vi "Teleop.vi"(10 "Match Info":T1={"Autonomous Elapsed Seconds"=0.0, "TeleOp Elapsed Seconds"=0.0, "Disabled Elapsed Seconds"=0.0, "Visited Autonomous"=FALSE, "Visited TeleOp"=FALSE, "Visited Disabled"=FALSE, "Autonomous Settings"={"Autonomous Style"=enum."Independent", "VI Refnum"=refnum}}, 11 "Call Context":T2) -> ()   [LabVIEW 2019]
doc: "This VI is called for each TeleOp packet received from the DS where the robot is not disabled. It is often used to read from the joysticks and update I/O or to update setpoints for timed control loops. It should complete and return within 20 milliseconds or it may miss DS packets."
uses:
  <vilib>/Rock Robotics/WPI/DriverStation/WPI_DriverStationDerivedRobotMode.ctl
  <vilib>/Rock Robotics/WPI/DriverStation/WPI_DriverStationMatch Info.ctl
  <vilib>/Rock Robotics/WPI/DriverStation/WPI_DriverStationRobotMode2.ctl
  <vilib>/Rock Robotics/WPI/ThirdParty/REV Robotics/SPARK MAX/Typedef/Spark MAX Control Type.ctl
  <vilib>/Rock Robotics/WPI/Utilities/WPI_GetSetVariantRefNum.vi
  Robot Global Data.vi
  <vilib>/Rock Robotics/Network Tables/NT Write Number.vi
  <vilib>/Rock Robotics/Network Tables/NT Write Boolean.vi
  <vilib>/Rock Robotics/WPI/RobotDrive/WPI_RobotDriveArcadeDrive_Standard(NoSaturation).vi
  <vilib>/Rock Robotics/Network Tables/NT Write Numeric Array.vi
panel:
  in  "error in":errorcluster
  # "Click here to set min"
  # "Click here to set max"
  # "Click here to set min"
  # "Click here to set max"
  # "Click here to set min"
  # "Click here to set max"
  # "Click here to set min"
  # "Click here to set max"
  # "Click here to set min"
  # "Click here to set max"
  # "Click here to set min"
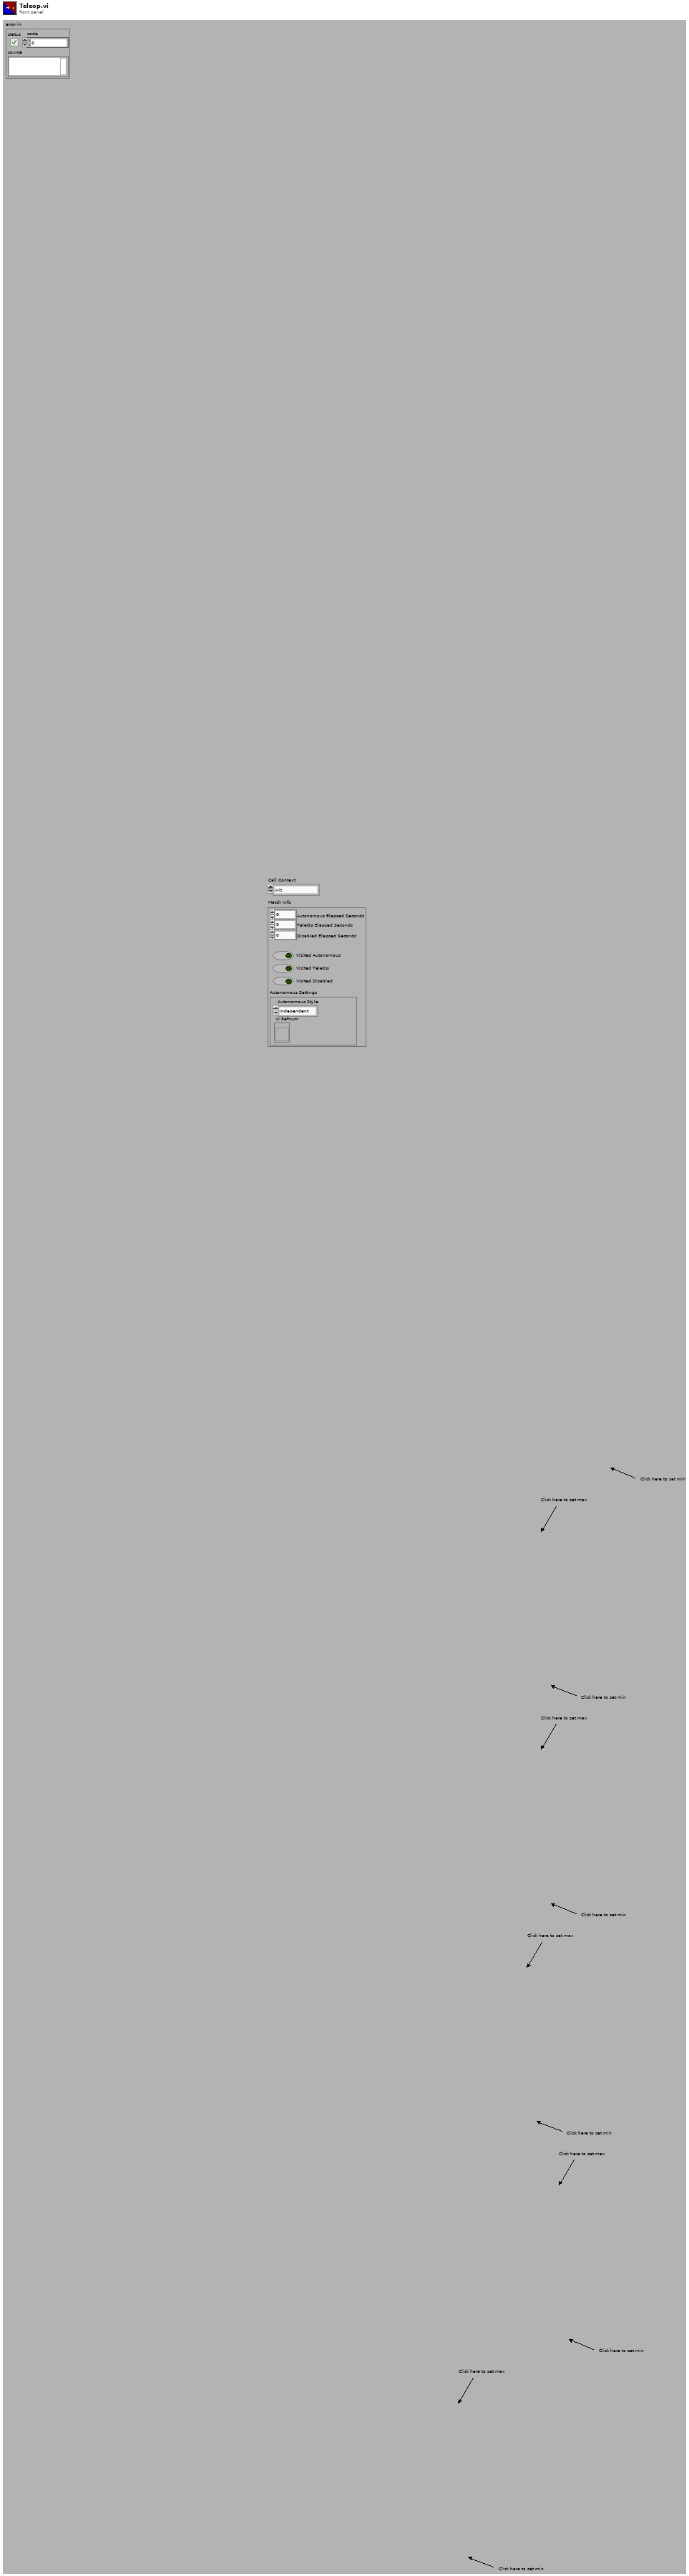
[diagram p1: front panel]
types:
  T1 = typedef "WPI_DriverStationMatch Info.ctl" = cluster{"Autonomous Elapsed Seconds":dbl, "TeleOp Elapsed Seconds":dbl, "Disabled Elapsed Seconds":dbl, "Visited Autonomous":bool, "Visited TeleOp":bool, "Visited Disabled":bool, "Autonomous Settings":cluster{"Autonomous Style":enum16{"Iterative", "Independent"}, "VI Refnum":refnum<vi>}}
  T2 = typedef "WPI_DriverStationDerivedRobotMode.ctl" = enum16{"Init", "Execute", "Stop"}
  T3 = typedef "WPI_JoystickDevRef.ctl" = cluster{"Device":T4}
  T4 = typedef "WPI_JoystickDeviceEnum.ctl" = enum16{"USB 0", "USB 1", "USB 2", "USB 3", "USB 4", "USB 5"}
  T5 = typedef "WPI_MotorControlDeviceRef.ctl" = cluster{"DeviceStatus":errorcluster, "Type":T6, "PWM":cluster{"PWM Channel":T7, "DeadBand":T8}, "CAN":cluster{"Device Number":u8, "SetOutput VI Ref":variant, "GetOutput VI Ref":variant, "Enable VI Ref":variant, "Disable VI Ref":variant, "Data":variant}, "Invert":bool, "DIO PWM":cluster{"PWM \"Enable\" Channel":T7, "DIOChannel":T9, "PWM Rate":dbl}}
  T6 = typedef "WPI_MotorControlType.ctl" = enum16{"PWM", "CAN", "DIO PWM"}
  T7 = typedef "FPGA_DIOPWMChannel.ctl" = enum8{"PWM 0", "PWM 1", "PWM 2", "PWM 3", "PWM 4", "PWM 5", "PWM 6", "PWM 7", "PWM 8", "PWM 9", "PWM MXP 0", "PWM MXP 1", "PWM MXP 2", "PWM MXP 3", "PWM MXP 4", "PWM MXP 5", "PWM MXP 6", "PWM MXP 7", "PWM MXP 8", "PWM MXP 9", "Invalid"}
  T8 = typedef "WPI_PWMDeadband.ctl" = cluster{"Name":string, "maxPositivePwm":i32, "minPositivePwm":i32, "centerPwm":i32, "maxNegativePwm":i32, "minNegativePwm":i32, "angularRange":u16}
  T9 = typedef "FPGA_DIOChannel.ctl" = enum8{"DIO 0", "DIO 1", "DIO 2", "DIO 3", "DIO 4", "DIO 5", "DIO 6", "DIO 7", "DIO 8", "DIO 9", "DIO MXP 0", "DIO MXP 1", "DIO MXP 2", "DIO MXP 3", "DIO MXP 4", "DIO MXP 5", "DIO MXP 6", "DIO MXP 7", "DIO MXP 8", "DIO MXP 9", "DIO MXP 10", "DIO MXP 11", "DIO MXP 12", "DIO MXP 13", "DIO MXP 14", "DIO MXP 15", "SPI Port CS1", "SPI Port CS2", "SPI Port CS3", "SPI Port MISO", "SPI Port MOSI", "Invalid"}
  T10 = typedef "WPI_RobotDriveDevRef.ctl" = cluster{"DevStatus":errorcluster, "Motors[]":T5[], "Square Inputs":bool, "Max Output":dbl}
  T11 = typedef "WPI_ServoDeviceRef.ctl" = cluster{"DeviceStatus":errorcluster, "PWM Channel":T7, "DeadBand":T8}
  T12 = typedef "Spark MAX Control Type.ctl" = enum16{"Percent VBus", "Voltage", "Velocity", "Position", "Smart Motion", "Current", "Smart Velocity"}
  T13 = typedef "WPI_DriverStationRobotMode2.ctl" = enum16{"Autonomous Disabled", "Autonomous Enabled", "Teleop Disabled", "Teleop Enabled", "Disconnected", "Finish", "Test Disabled", "Test Enabled", "Emergency Stopped"}
  T14 = cluster{"P Gain":dbl, "I Gain":dbl, "D Gain":dbl, "F Gain":dbl, "I Zone":dbl, "Min Output":dbl, "Max Output":dbl}
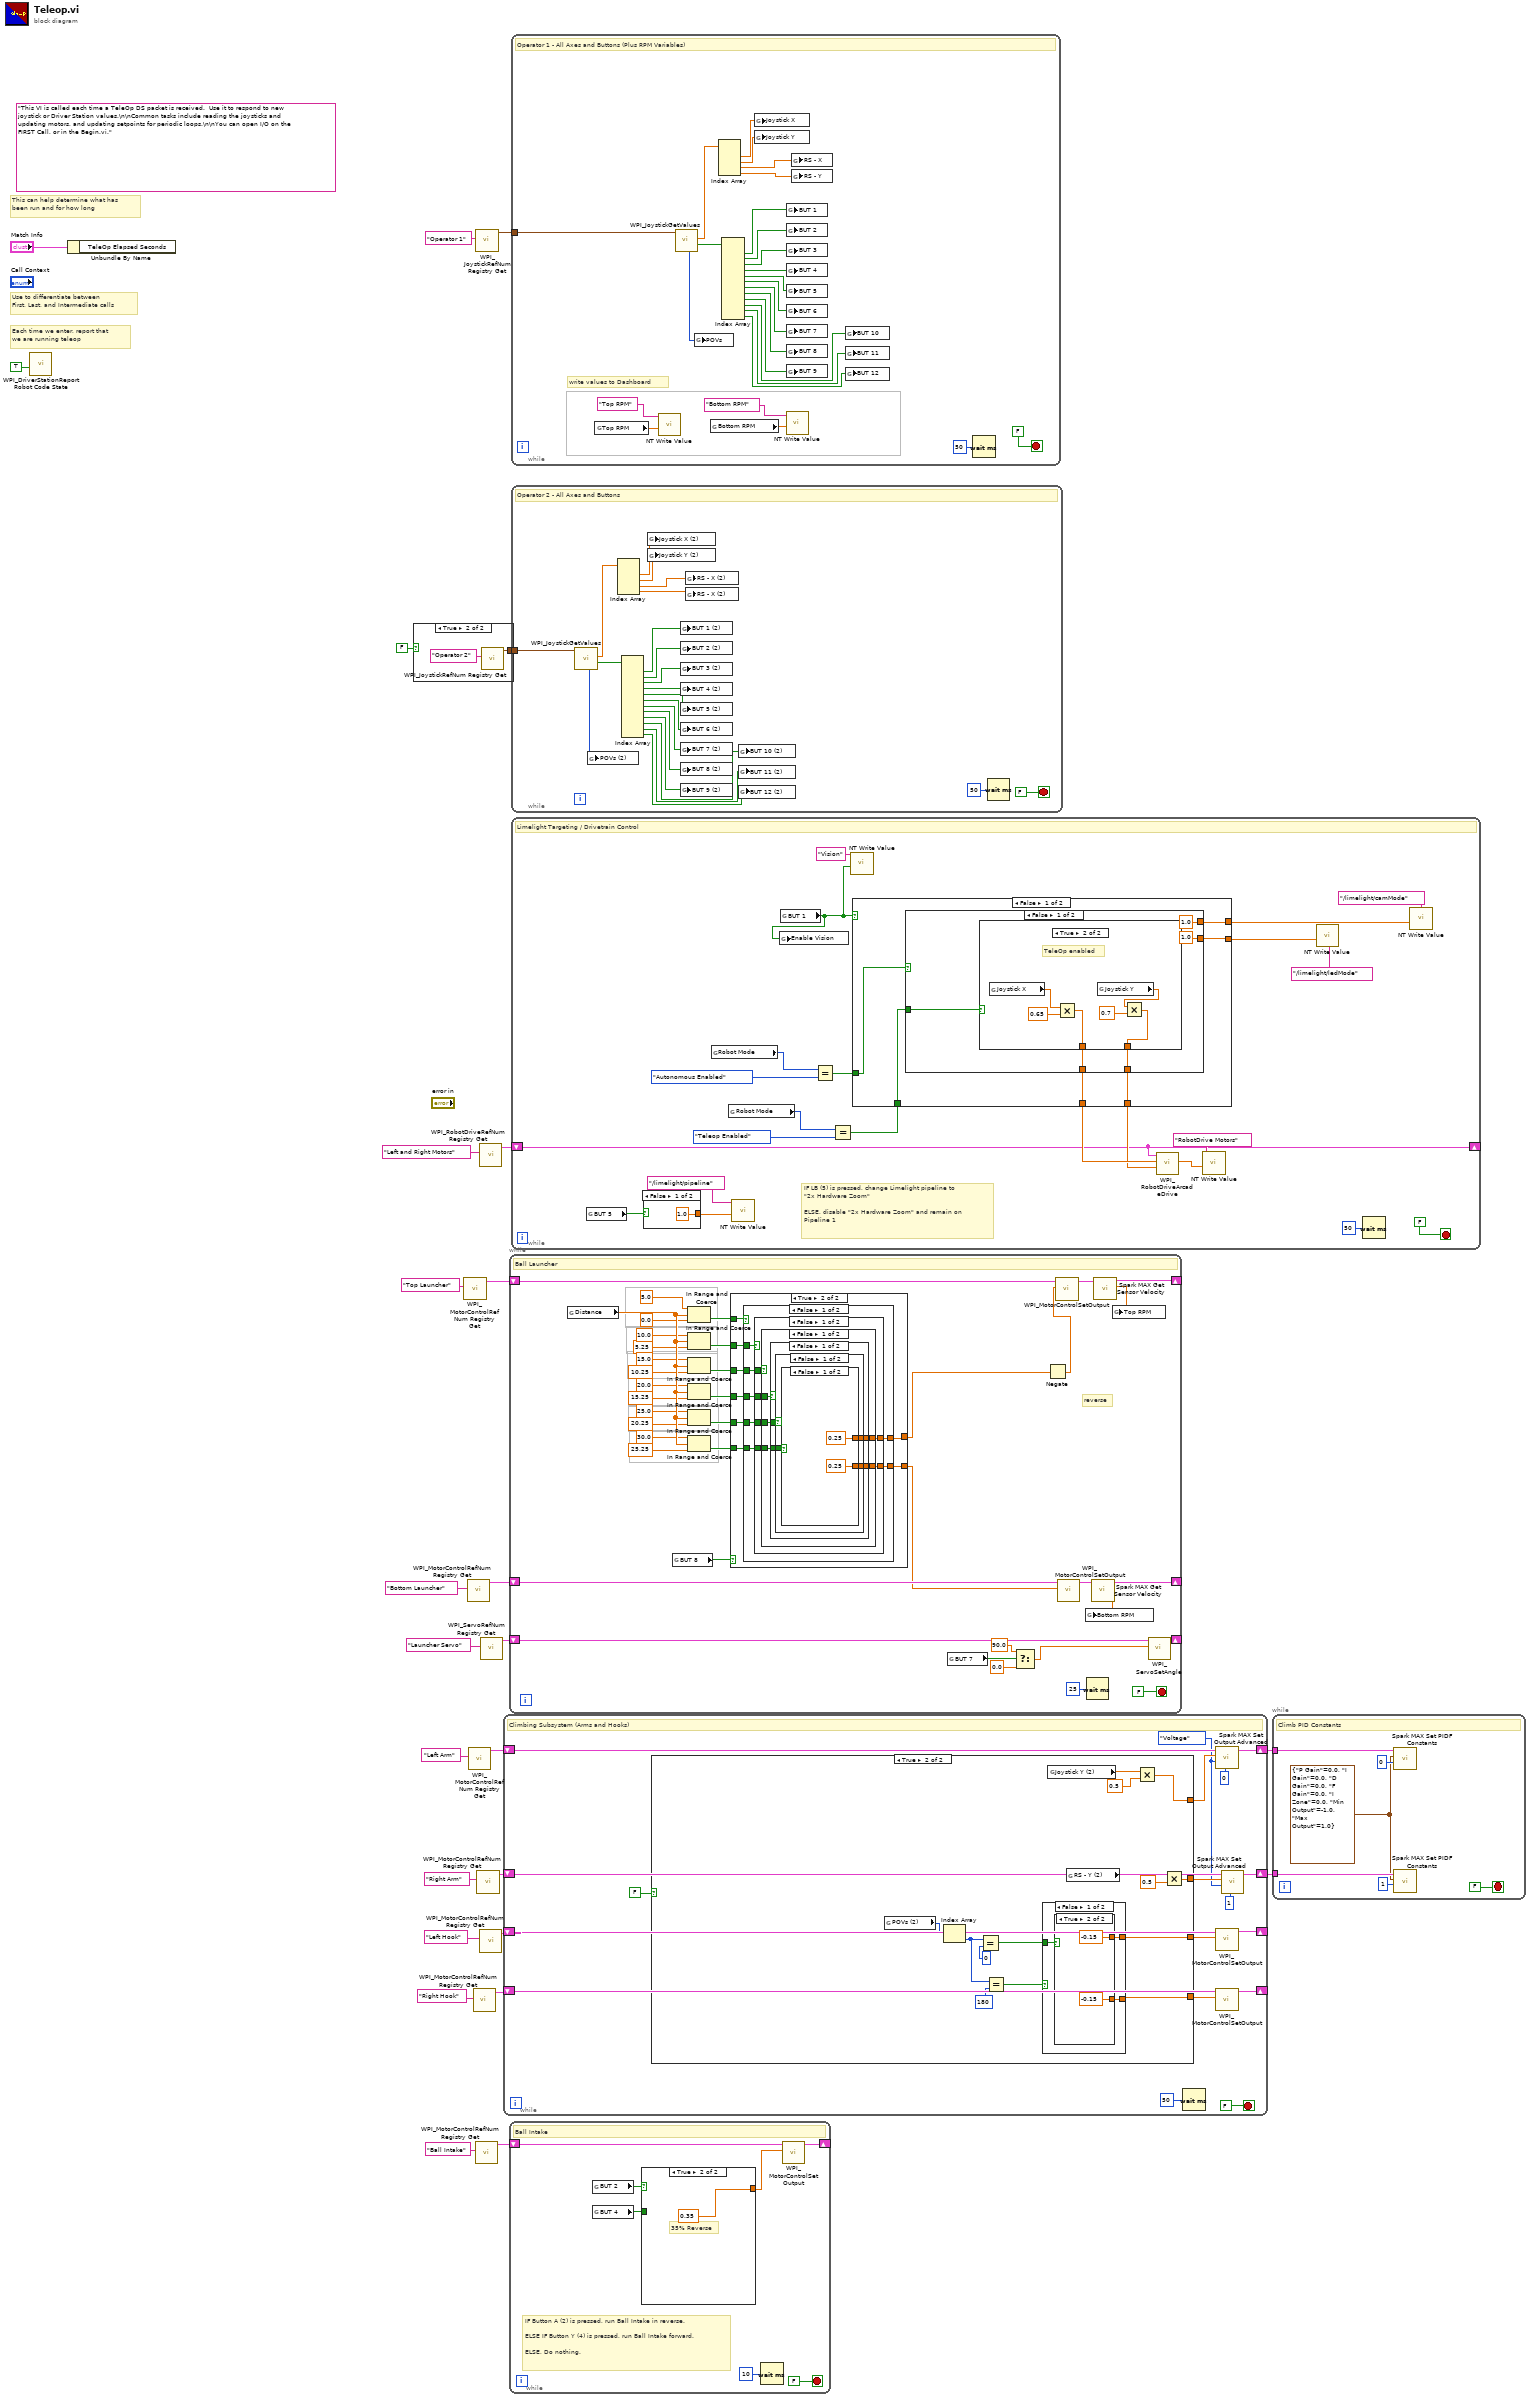
[diagram p0: block diagram]
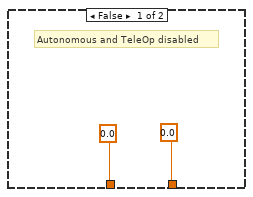
[diagram p3: hidden frame]
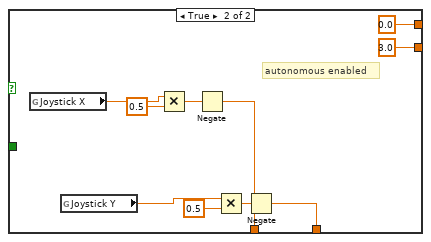
[diagram p4: hidden frame]
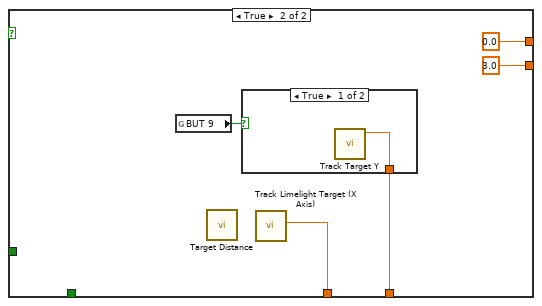
[diagram p5: hidden frame]
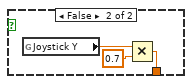
[diagram p6: hidden frame]
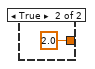
[diagram p7: hidden frame]
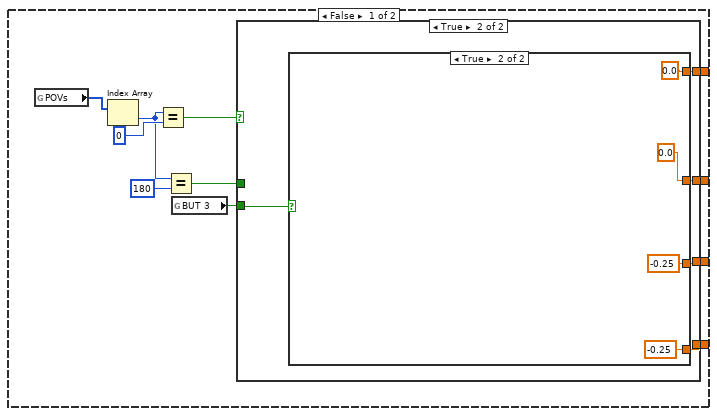
[diagram p8: hidden frame]
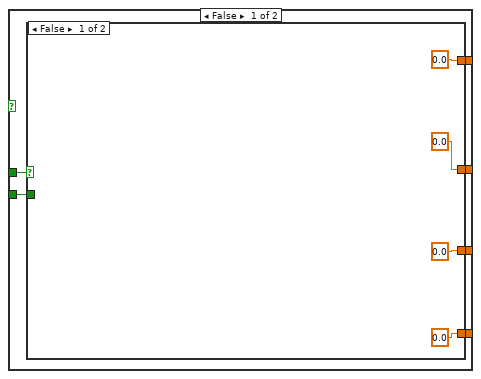
[diagram p9: hidden frame]
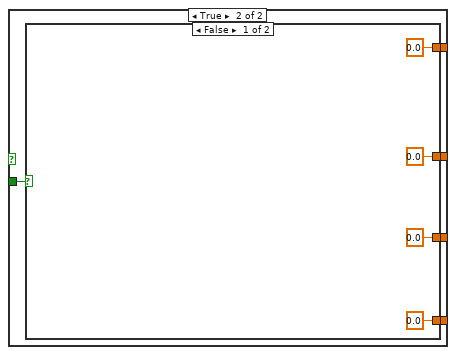
[diagram p10: hidden frame]
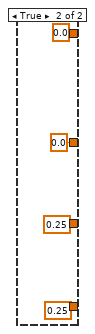
[diagram p11: hidden frame]
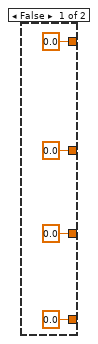
[diagram p12: hidden frame]
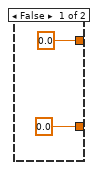
[diagram p13: hidden frame]
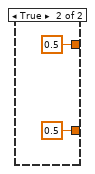
[diagram p14: hidden frame]
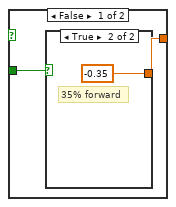
[diagram p15: hidden frame]
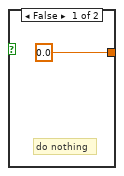
[diagram p16: hidden frame]
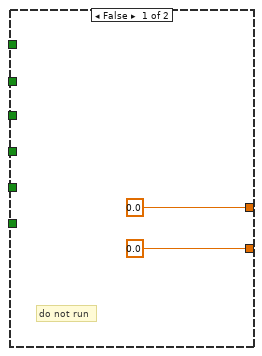
[diagram p17: hidden frame]
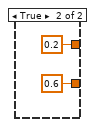
[diagram p18: hidden frame]
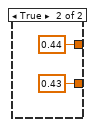
[diagram p19: hidden frame]
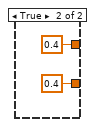
[diagram p20: hidden frame]
diagram:
  (unwired) "This VI is called each time a TeleOp DS packet is received.  Use it to respond to new joystick or Driver Station values.\n\nCommon tasks include reading the joysticks and updating motors, and updating setpoints for periodic loops.\n\nYou can open I/O on the FIRST Call, or in the Begin.vi."
  # "Each time we enter, report that\nwe are running teleop"
  # "Use to differentiate between\nFirst, Last, and Intermediate calls"
  # "This can help determine what has\nbeen run and for how long"
  n1 = call <vilib>:"WPI_DriverStationReport Robot Code State.vi"("TeleOp"=TRUE ("Autonomous")) -> ()  [unwired: 10 in, 1 out]
  n2 = Unbundle By Name("Match Info") -> ()  [unwired: 1 out]
  n3 = case shown="True" FALSE {
    tunnel: [_ w27] -> w8
    frame False {
    }
    frame True {
      n4 = call <vilib>:"WPI_JoystickRefNum Registry Get.vi"("refnum name"="Operator 2") -> ("JoystickDevRef"=w27:T3)  [unwired: 1 in, 9 out]
    }
  }
  n5 = call <vilib>:"WPI_MotorControlRefNum Registry Get.vi"("refnum name"="Top Launcher") -> ("MotorControlDevRef"=w20:T5)  [unwired: 9 in, 1 out]
  n6 = call <vilib>:"WPI_MotorControlRefNum Registry Get.vi"("refnum name"="Bottom Launcher") -> ("MotorControlDevRef"=w22:T5)  [unwired: 9 in, 1 out]
  n7 = call <vilib>:"WPI_MotorControlRefNum Registry Get.vi"("refnum name"="Left Arm") -> ("MotorControlDevRef"=w14:T5)  [unwired: 9 in, 1 out]
  n8 = call <vilib>:"WPI_MotorControlRefNum Registry Get.vi"("refnum name"="Right Hook") -> ("MotorControlDevRef"=w11:T5)  [unwired: 9 in, 1 out]
  n9 = call <vilib>:"WPI_MotorControlRefNum Registry Get.vi"("refnum name"="Ball Intake") -> ("MotorControlDevRef"=w16:T5)  [unwired: 9 in, 1 out]
  n10 = call <vilib>:"WPI_JoystickRefNum Registry Get.vi"("refnum name"="Operator 1") -> ("JoystickDevRef"=w7:T3)  [unwired: 1 in, 9 out]
  n11 = call <vilib>:"WPI_MotorControlRefNum Registry Get.vi"("refnum name"="Right Arm") -> ("MotorControlDevRef"=w13:T5)  [unwired: 9 in, 1 out]
  n12 = call <vilib>:"WPI_RobotDriveRefNum Registry Get.vi"("refnum name"="Left and Right Motors") -> ("RobotDriveDevRef"=w1:T10)  [unwired: 1 in, 9 out]
  n13 = call <vilib>:"WPI_MotorControlRefNum Registry Get.vi"("refnum name"="Left Hook") -> ("MotorControlDevRef"=w12:T5)  [unwired: 9 in, 1 out]
  n14 = call <vilib>:"WPI_ServoRefNum Registry Get.vi"("refnum name"="Launcher Servo") -> ("ServoDeviceRef"=w18:T11)  [unwired: 9 in, 1 out]
  n15 = while {
    shift-right: [w45] -> w3
    shift-left: w14 -> [w44]
    shift-right: [w33] -> w2
    shift-left: w13 -> [w32]
    shift-right: [w41] -> _
    shift-left: w11 -> [w40]
    shift-right: [w42] -> _
    shift-left: w12 -> [w39]
    stop <- FALSE stop-if-true
    w29 = Spark_MAX_Control_Type."Voltage" ("Control Mode")
    # "Climbing Subsystem (Arms and Hooks)"
    n16 = case shown="True" FALSE {
      tunnel: [w56 w107] -> w38
      tunnel: [w57 w106] -> w37
      tunnel: [w54 w100] -> w36
      tunnel: [w55 w99] -> w31
      frame False {
        n17 = global read "Robot Global Data.vi" "POVs"() -> (w53:i16[])
        n18 = Index Array(array=w53) -> (element=w51:i16)  [unwired: 1 in]
        n19 = Equal?(x=w51, y=i16 0) -> (x = y?=w49:bool)
        n20 = Equal?(x=w51, y=i16 180) -> (x = y?=w48:bool)
        n21 = global read "Robot Global Data.vi" "BUT 3"() -> (w47:bool)
        n22 = case shown="True" w49 {
          tunnel: [w63 w82] -> w57
          tunnel: [w62 w81] -> w56
          tunnel: [w61 w83] -> w55
          tunnel: [w60 w84] -> w54
          tunnel: w48 -> [w59 _]
          tunnel: w47 -> [w58 w85]
          frame False {
            n23 = case shown="False" w59 {
              tunnel: [0.0 ("Output") w72] -> w63
              tunnel: [0.0 ("Output") w71] -> w62
              tunnel: [0.0 w70] -> w61
              tunnel: [0.0 w69] -> w60
              tunnel: w58 -> [_ w68]
              frame False {
              }
              frame True {
                n24 = case shown="False" w68 {
                  tunnel: [0.0 ("Output") 0.25 ("Output")] -> w72
                  tunnel: [0.0 ("Output") 0.25 ("Output")] -> w71
                  tunnel: [0.0 0.0] -> w70
                  tunnel: [0.0 0.0] -> w69
                  frame False {
                  }
                  frame True {
                  }
                }
              }
            }
          }
          frame True {
            n25 = case shown="True" w85 {
              tunnel: [0.0 0.0] -> w84
              tunnel: [0.0 0.0] -> w83
              tunnel: [0.0 ("Output") -0.25 ("Output")] -> w82
              tunnel: [0.0 ("Output") -0.25 ("Output")] -> w81
              frame False {
              }
              frame True {
              }
            }
          }
        }
      }
      frame True {
        n26 = global read "Robot Global Data.vi" "POVs (2)"() -> (w105:i16[])
        n27 = Index Array(array=w105) -> (element=w104:i16)  [unwired: 1 in]
        n28 = Equal?(x=w104, y=i16 0) -> (x = y?=w101:bool)
        n29 = Equal?(x=w104, y=i16 180) -> (x = y?=w102:bool)
        n30 = case shown="False" w102 {
          tunnel: [w110 0.5 ("Output")] -> w107
          tunnel: [w109 0.5 ("Output")] -> w106
          tunnel: w101 -> [w108 _]
          frame False {
            n31 = case shown="True" w108 {
              tunnel: [0.0 ("Output") -0.15 ("Output")] -> w110
              tunnel: [0.0 ("Output") -0.15 ("Output")] -> w109
              frame False {
              }
              frame True {
              }
            }
          }
          frame True {
          }
        }
        n32 = global read "Robot Global Data.vi" "Joystick Y (2)"() -> (w98:dbl)
        n33 = global read "Robot Global Data.vi" "RS - Y (2)"() -> (w97:dbl)
        n34 = Multiply(x=w98, y=0.5) -> (x*y=w100:dbl)
        n35 = Multiply(x=w97, y=0.5) -> (x*y=w99:dbl)
      }
    }
    n36 = Wait (ms)(milliseconds to wait=u32 50) -> ()  [unwired: 1 out]
    n37 = call <vilib>:"Spark MAX Set Output Advanced.vi"("PIDF Slot (0)"=0, "Control Mode"=w29, "Setpoint"=w36, "MotorControlDevRef"=w44) -> ("MotorControlDevRef"=w45:T5)  [unwired: 6 in, 1 out]
    n38 = call <vilib>:"WPI_MotorControlSetOutput.vi"("Output"=w37, "MotorControlDevRef"=w39) -> ("MotorControlDevRef"=w42:T5)  [unwired: 7 in, 2 out]
    n39 = call <vilib>:"WPI_MotorControlSetOutput.vi"("Output"=w38, "MotorControlDevRef"=w40) -> ("MotorControlDevRef"=w41:T5)  [unwired: 7 in, 2 out]
    n40 = call <vilib>:"Spark MAX Set Output Advanced.vi"("PIDF Slot (0)"=1, "Control Mode"=w29, "Setpoint"=w31, "MotorControlDevRef"=w32) -> ("MotorControlDevRef"=w33:T5)  [unwired: 6 in, 1 out]
  }
  n41 = while {
    shift-right: [w147] -> _
    shift-left: w22 -> [w148]
    shift-right: [w145] -> _
    shift-left: w20 -> [w146]
    shift-right: [w144] -> _
    shift-left: w18 -> [w139]
    stop <- FALSE stop-if-true
    # "reverse"
    # "Ball Launcher"
    n42 = global read "Robot Global Data.vi" "Distance"() -> (w138:dbl)
    n43 = global read "Robot Global Data.vi" "BUT 8"() -> (w119:bool)
    n44 = In Range and Coerce(upper limit=5.0, x=w138, lower limit=0.0) -> (In Range?=w137:bool)  [unwired: 1 out]
    n45 = In Range and Coerce(upper limit=10.0, x=w138, lower limit=5.25) -> (In Range?=w136:bool)  [unwired: 1 out]
    n46 = In Range and Coerce(upper limit=15.0, x=w138, lower limit=10.25) -> (In Range?=w120:bool)  [unwired: 1 out]
    n47 = In Range and Coerce(upper limit=20.0, x=w138, lower limit=15.25) -> (In Range?=w121:bool)  [unwired: 1 out]
    n48 = In Range and Coerce(upper limit=25.0, x=w138, lower limit=20.25) -> (In Range?=w122:bool)  [unwired: 1 out]
    n49 = In Range and Coerce(upper limit=30.0, x=w138, lower limit=25.25) -> (In Range?=w123:bool)  [unwired: 1 out]
    n50 = case shown="True" w119 {
      tunnel: [0.0 ("Output") w159] -> w118
      tunnel: [0.0 ("Output") w158] -> w117
      tunnel: w137 -> [_ w165]
      tunnel: w120 -> [_ w163]
      tunnel: w121 -> [_ w162]
      tunnel: w122 -> [_ w161]
      tunnel: w123 -> [_ w160]
      tunnel: w136 -> [_ w164]
      frame False {
        # "do not run"
      }
      frame True {
        n51 = case shown="False" w165 {
          tunnel: w164 -> [w172 _]
          tunnel: w163 -> [w171 _]
          tunnel: w162 -> [w170 _]
          tunnel: w161 -> [w169 _]
          tunnel: w160 -> [w168 _]
          tunnel: [w167 0.0 ("Output")] -> w159
          tunnel: [w166 0.0 ("Output")] -> w158
          frame False {
            n52 = case shown="False" w172 {
              tunnel: w171 -> [w178 _]
              tunnel: w170 -> [w177 _]
              tunnel: w169 -> [w176 _]
              tunnel: w168 -> [w175 _]
              tunnel: [w174 0.4 ("Output")] -> w167
              tunnel: [w173 0.65 ("Output")] -> w166
              frame False {
                n53 = case shown="False" w178 {
                  tunnel: w177 -> [w183 _]
                  tunnel: w176 -> [w182 _]
                  tunnel: w175 -> [w181 _]
                  tunnel: [w180 0.3 ("Output")] -> w174
                  tunnel: [w179 0.55 ("Output")] -> w173
                  frame False {
                    n54 = case shown="False" w183 {
                      tunnel: w182 -> [w187 _]
                      tunnel: w181 -> [w186 _]
                      tunnel: [w185 0.4 ("Output")] -> w180
                      tunnel: [w184 0.4 ("Output")] -> w179
                      frame False {
                        n55 = case shown="False" w187 {
                          tunnel: w186 -> [w190 _]
                          tunnel: [w189 0.44 ("Output")] -> w185
                          tunnel: [w188 0.43 ("Output")] -> w184
                          frame False {
                            n56 = case shown="False" w190 {
                              tunnel: [0.25 ("Output") 0.2 ("Output")] -> w189
                              tunnel: [0.25 ("Output") 0.6 ("Output")] -> w188
                              frame False {
                              }
                              frame True {
                              }
                            }
                          }
                          frame True {
                          }
                        }
                      }
                      frame True {
                      }
                    }
                  }
                  frame True {
                  }
                }
              }
              frame True {
              }
            }
          }
          frame True {
            # "do not run"
          }
        }
      }
    }
    n57 = global read "Robot Global Data.vi" "BUT 7"() -> (w143:bool)
    n58 = Select(t=90.0, s=w143, f=0.0) -> (s? t:f=w140:dbl)
    n59 = Negate(x=w118) -> (-x=w155:dbl)
    n60 = call <vilib>:"WPI_MotorControlSetOutput.vi"("Output"=w155, "MotorControlDevRef"=w146) -> ("MotorControlDevRef"=w153:T5)  [unwired: 7 in, 2 out]
    n61 = call <vilib>:"WPI_MotorControlSetOutput.vi"("Output"=w117, "MotorControlDevRef"=w148) -> ("MotorControlDevRef"=w154:T5)  [unwired: 7 in, 2 out]
    n62 = Wait (ms)(milliseconds to wait=u32 25) -> ()  [unwired: 1 out]
    n63 = call <vilib>:"Spark MAX Get Sensor Velocity.vi"("MotorControlDevRef in"=w154) -> ("Sensor Velocity"=w152:dbl, "MotorControlDevRef out"=w147:T5)  [unwired: 7 in, 2 out]
    n64 = global write "Robot Global Data.vi" "Bottom RPM"(w152) -> ()
    n65 = call <vilib>:"Spark MAX Get Sensor Velocity.vi"("MotorControlDevRef in"=w153) -> ("Sensor Velocity"=w151:dbl, "MotorControlDevRef out"=w145:T5)  [unwired: 7 in, 2 out]
    n66 = global write "Robot Global Data.vi" "Top RPM"(w151) -> ()
    n67 = call <vilib>:"WPI_ServoSetAngle.vi"("Angle"=w140, "ServoDeviceRef"=w139) -> ("ServoDeviceRef"=w144:T11)  [unwired: 8 in, 1 out]
  }
  n68 = while {
    shift-right: [w208] -> _
    shift-left: w16 -> [w209]
    stop <- FALSE stop-if-true
    # "IF Button A (2) is pressed, run Ball Intake in reverse. \n\nELSE IF Button Y (4) is pressed, run Ball Intake forward.\n\nELSE, Do nothing."
    # "Ball Intake"
    n69 = global read "Robot Global Data.vi" "BUT 2"() -> (w206:bool)
    n70 = global read "Robot Global Data.vi" "BUT 4"() -> (w207:bool)
    n71 = case shown="True" w206 {
      tunnel: [w213 0.35 ("Output")] -> w205
      tunnel: w207 -> [w212 _]
      frame False {
        n72 = case shown="True" w212 {
          tunnel: [0.0 ("Output") -0.35 ("Output")] -> w213
          frame False {
            # "do nothing"
          }
          frame True {
            # "35% forward"
          }
        }
      }
      frame True {
        # "35% Reverse"
      }
    }
    n73 = Wait (ms)(milliseconds to wait=u32 10) -> ()  [unwired: 1 out]
    n74 = call <vilib>:"WPI_MotorControlSetOutput.vi"("Output"=w205, "MotorControlDevRef"=w209) -> ("MotorControlDevRef"=w208:T5)  [unwired: 7 in, 2 out]
  }
  n75 = while {
    tunnel: w7 -> [w219]
    stop <- FALSE stop-if-true
    # "write values to Dashboard"
    # "Operator 1 - All Axes and Buttons (Plus RPM Variables)"
    n76 = global read "Robot Global Data.vi" "Top RPM"() -> (w224:dbl)
    n77 = call-poly <vilib>:"NT Write Value.vi"("Numeric"=w224, "Name"="Top RPM") -> ()  [unwired: 9 in, 1 out]
    n78 = call <vilib>:"WPI_JoystickGetValues.vi"("JoystickDevRef"=w219) -> ("Buttons"=w241:bool[], "Axes"=w228:dbl[], "POVs"=w220:i16[])  [unwired: 6 in, 2 out]
    n79 = global write "Robot Global Data.vi" "POVs"(w220) -> ()
    n80 = global read "Robot Global Data.vi" "Bottom RPM"() -> (w222:dbl)
    n81 = Index Array(array=w228) -> (element #1=w218:dbl, element #2=w217:dbl, element #3=w221:dbl, element #4=w227:dbl)  [unwired: 4 in]
    n82 = Index Array(array=w241) -> (element #1=w240:bool, element #2=w239:bool, element #3=w238:bool, element #4=w237:bool, element #5=w236:bool, element #6=w235:bool, element #7=w234:bool, element #8=w233:bool, element #9=w232:bool, element #10=w231:bool, element #11=w230:bool, element #12=w229:bool)  [unwired: 12 in]
    n83 = global write "Robot Global Data.vi" "Joystick X"(w218) -> ()
    n84 = global write "Robot Global Data.vi" "Joystick Y"(w217) -> ()
    n85 = call-poly <vilib>:"NT Write Value.vi"("Numeric"=w222, "Name"="Bottom RPM") -> ()  [unwired: 9 in, 1 out]
    n86 = global write "Robot Global Data.vi" "BUT 1"(w240) -> ()
    n87 = global write "Robot Global Data.vi" "BUT 2"(w239) -> ()
    n88 = global write "Robot Global Data.vi" "BUT 3"(w238) -> ()
    n89 = global write "Robot Global Data.vi" "BUT 4"(w237) -> ()
    n90 = global write "Robot Global Data.vi" "BUT 5"(w236) -> ()
    n91 = global write "Robot Global Data.vi" "BUT 6"(w235) -> ()
    n92 = global write "Robot Global Data.vi" "BUT 7"(w234) -> ()
    n93 = global write "Robot Global Data.vi" "BUT 8"(w233) -> ()
    n94 = global write "Robot Global Data.vi" "BUT 9"(w232) -> ()
    n95 = global write "Robot Global Data.vi" "RS - X"(w221) -> ()
    n96 = global write "Robot Global Data.vi" "RS - Y"(w227) -> ()
    n97 = global write "Robot Global Data.vi" "BUT 10"(w231) -> ()
    n98 = global write "Robot Global Data.vi" "BUT 11"(w230) -> ()
    n99 = global write "Robot Global Data.vi" "BUT 12"(w229) -> ()
    n100 = Wait (ms)(milliseconds to wait=u32 50) -> ()  [unwired: 1 out]
  }
  n101 = while {
    tunnel: w8 -> [w248]
    stop <- FALSE stop-if-true
    # "Operator 2 - All Axes and Buttons"
    n102 = call <vilib>:"WPI_JoystickGetValues.vi"("JoystickDevRef"=w248) -> ("Buttons"=w250:bool[], "Axes"=w247:dbl[], "POVs"=w249:i16[])  [unwired: 6 in, 2 out]
    n103 = global write "Robot Global Data.vi" "POVs (2)"(w249) -> ()
    n104 = Index Array(array=w247) -> (element #1=w246:dbl, element #2=w245:dbl, element #3=w244:dbl, element #4=w243:dbl)  [unwired: 4 in]
    n105 = Index Array(array=w250) -> (element #1=w251:bool, element #2=w252:bool, element #3=w253:bool, element #4=w254:bool, element #5=w255:bool, element #6=w256:bool, element #7=w257:bool, element #8=w258:bool, element #9=w259:bool, element #10=w260:bool, element #11=w261:bool, element #12=w262:bool)  [unwired: 12 in]
    n106 = global write "Robot Global Data.vi" "Joystick X (2)"(w246) -> ()
    n107 = global write "Robot Global Data.vi" "Joystick Y (2)"(w245) -> ()
    n108 = global write "Robot Global Data.vi" "BUT 1 (2)"(w251) -> ()
    n109 = global write "Robot Global Data.vi" "BUT 2 (2)"(w252) -> ()
    n110 = global write "Robot Global Data.vi" "BUT 3 (2)"(w253) -> ()
    n111 = global write "Robot Global Data.vi" "BUT 4 (2)"(w254) -> ()
    n112 = global write "Robot Global Data.vi" "BUT 5 (2)"(w255) -> ()
    n113 = global write "Robot Global Data.vi" "BUT 6 (2)"(w256) -> ()
    n114 = global write "Robot Global Data.vi" "BUT 7 (2)"(w257) -> ()
    n115 = global write "Robot Global Data.vi" "BUT 8 (2)"(w258) -> ()
    n116 = global write "Robot Global Data.vi" "BUT 9 (2)"(w259) -> ()
    n117 = global write "Robot Global Data.vi" "RS - X (2)"(w244) -> ()
    n118 = global write "Robot Global Data.vi" "RS - X (2)"(w243) -> ()
    n119 = global write "Robot Global Data.vi" "BUT 10 (2)"(w260) -> ()
    n120 = global write "Robot Global Data.vi" "BUT 11 (2)"(w261) -> ()
    n121 = global write "Robot Global Data.vi" "BUT 12 (2)"(w262) -> ()
    n122 = Wait (ms)(milliseconds to wait=u32 50) -> ()  [unwired: 1 out]
  }
  n123 = while {
    shift-right: [w267] -> _
    shift-left: w1 -> [w267]
    stop <- FALSE stop-if-true
    # "IF LB (5) is pressed, change Limelight pipeline to \n\"2x Hardware Zoom\"\n\nELSE, disable \"2x Hardware Zoom\" and remain on\nPipeline 1"
    # "Limelight Targeting / Drivetrain Control"
    n124 = global read "Robot Global Data.vi" "BUT 5"() -> (w270:bool)
    n125 = case shown="False" w270 {
      tunnel: [1.0 ("Numeric") 2.0 ("Numeric")] -> w283
      frame False {
      }
      frame True {
      }
    }
    n126 = global read "Robot Global Data.vi" "Robot Mode"() -> (w278:T13)
    n127 = global read "Robot Global Data.vi" "Robot Mode"() -> (w274:T13)
    n128 = call-poly <vilib>:"NT Write Value.vi"("Numeric"=w283, "Name"="/limelight/pipeline") -> ()  [unwired: 9 in, 1 out]
    n129 = global read "Robot Global Data.vi" "BUT 1"() -> (w265:bool)
    n130 = global write "Robot Global Data.vi" "Enable Vision"(w265) -> ()
    n131 = Equal?(x=w278, y=WPI_DriverStationRobotMode2."Autonomous Enabled") -> (x = y?=w276:bool)
    n132 = Equal?(x=w274, y=WPI_DriverStationRobotMode2."Teleop Enabled") -> (x = y?=w273:bool)
    n133 = call-poly <vilib>:"NT Write Value.vi"("Boolean"=w265, "Name"="Vision") -> ()  [unwired: 9 in, 1 out]
    n134 = case shown="False" w265 {
      tunnel: [w289 0.0 ("Numeric")] -> w280
      tunnel: [w288 3.0 ("Numeric")] -> w279
      tunnel: [w292 w318] -> w271
      tunnel: w276 -> [w290 _]
      tunnel: w273 -> [w291 _]
      tunnel: [w287 w317] -> w272
      frame False {
        n135 = case shown="False" w290 {
          tunnel: [w296 w315] -> w292
          tunnel: [w297 w314] -> w287
          tunnel: w291 -> [w295 _]
          tunnel: [1.0 ("Numeric") 0.0 ("Numeric")] -> w289
          tunnel: [1.0 ("Numeric") 3.0 ("Numeric")] -> w288
          frame False {
            n136 = case shown="True" w295 {
              tunnel: [0.0 ("Joystick X") w303] -> w297
              tunnel: [0.0 ("Joystick Y") w300] -> w296
              frame False {
                # "Autonomous and TeleOp disabled"
              }
              frame True {
                # "TeleOp enabled"
                n137 = global read "Robot Global Data.vi" "Joystick X"() -> (w305:dbl)
                n138 = Multiply(x=w305, y=0.65) -> (x*y=w303:dbl)
                n139 = global read "Robot Global Data.vi" "Joystick Y"() -> (w302:dbl)
                n140 = Multiply(x=w302, y=0.7) -> (x*y=w300:dbl)
              }
            }
          }
          frame True {
            # "autonomous enabled"
            n141 = global read "Robot Global Data.vi" "Joystick X"() -> (w310:dbl)
            n142 = global read "Robot Global Data.vi" "Joystick Y"() -> (w306:dbl)
            n143 = Multiply(x=w310, y=0.5) -> (x*y=w311:dbl)
            n144 = Negate(x=w311) -> (-x=w314:dbl)
            n145 = Multiply(x=w306, y=0.5) -> (x*y=w307:dbl)
            n146 = Negate(x=w307) -> (-x=w315:dbl)
          }
        }
      }
      frame True {
        n147 = global read "Robot Global Data.vi" "BUT 9"() -> (w316:bool)
        n148 = call "Target Distance.vi"() -> ()  [unwired: 12 in]
        n149 = case shown="True" w316 {
          tunnel: [w321 w324] -> w318
          frame True {
            n150 = call "Track Target Y.vi"() -> ("Joystick Y"=w321:dbl)  [unwired: 11 in]
          }
          frame False {
            n151 = global read "Robot Global Data.vi" "Joystick Y"() -> (w323:dbl)
            n152 = Multiply(x=w323, y=0.7) -> (x*y=w324:dbl)
          }
        }
        n153 = call "Track Limelight Target (X Axis).vi"() -> ("Joystick X"=w317:dbl)  [unwired: 11 in]
      }
    }
    n154 = call-poly <vilib>:"WPI_RobotDriveArcadeDrive.vi"("Y axis value"=w271, "X axis value"=w272, "RobotDriveDevRef"=w267) -> ("Motor Values"=w268:dbl[])  [unwired: 6 in, 2 out]
    n155 = call-poly <vilib>:"NT Write Value.vi"("Numeric Array"=w268, "Name"="RobotDrive Motors") -> ()  [unwired: 9 in, 1 out]
    n156 = call-poly <vilib>:"NT Write Value.vi"("Numeric"=w279, "Name"="/limelight/ledMode" ("LED Mode")) -> ()  [unwired: 9 in, 1 out]
    n157 = Wait (ms)(milliseconds to wait=u32 50) -> ()  [unwired: 1 out]
    n158 = call-poly <vilib>:"NT Write Value.vi"("Numeric"=w280, "Name"="/limelight/camMode" ("Camera Mode")) -> ()  [unwired: 9 in, 1 out]
  }
  n159 = while {
    tunnel: w3 -> [w331]
    tunnel: w2 -> [w329]
    stop <- FALSE stop-if-true
    w327 = T14 {"P Gain"=0.0, "I Gain"=0.0, "D Gain"=0.0, "F Gain"=0.0, "I Zone"=0.0, "Min Output"=-1.0, "Max Output"=1.0}
    # "Climb PID Constants"
    n160 = call <vilib>:"Spark MAX Set PIDF Constants.vi"("PIDF Slot"=0, "PID Constants"=w327, "MotorControlDeviceRef"=w331) -> ()  [unwired: 7 in, 2 out]
    n161 = call <vilib>:"Spark MAX Set PIDF Constants.vi"("PIDF Slot"=1, "PID Constants"=w327, "MotorControlDeviceRef"=w329) -> ()  [unwired: 7 in, 2 out]
  }
